vi "Append Two Strings - In Project.vi"(4 "String 2":string, 5 "String":string) -> (2 "String Measurement":string)   [LabVIEW 2010]
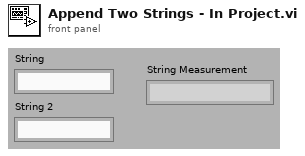
[diagram p1: front panel]
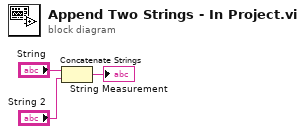
[diagram p0: block diagram]
diagram:
  n1 = Concatenate Strings("String", "String 2") -> (→"String Measurement":string)
